vi "Variables.vi"(8 "Channel":string[](array[string]), 10 "Test":string(combo), 11 "PMTs":string[](array[string])) -> (0 "Test":string, 2 "Channels":string[](array[string]), 3 "PMTs":string[](array[string]))   [LabVIEW 2018]
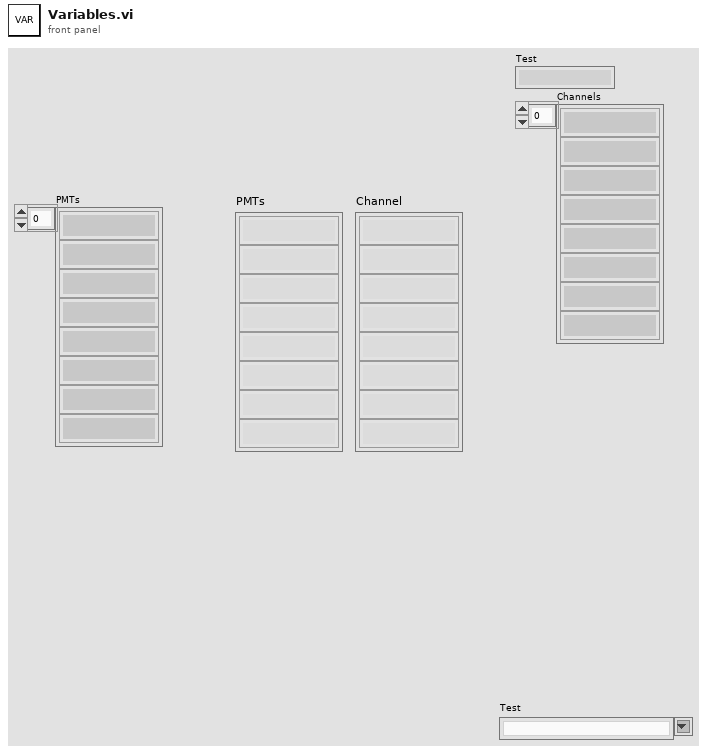
[diagram p1: front panel]
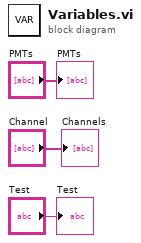
[diagram p0: block diagram]
diagram:
  "Test" <- "Test"
  "PMTs" <- "PMTs"
  "Channels" <- "Channel"
